vi "PI_Feedforward.vi"(5 "Motor Effort Axis":dbl[](array[numeric]) format="%_6g", 6 "dT":dbl, 7 "Position Axis":dbl[](array[numeric]) format="%_6g", 9 "Control Inputs":T2={"Kp"=0.01, "Ki"=0.0, "i upper"=0.0, "i lower"=0.0, "Output upper"=1.0, "Output lower"=-1.0}, 10 "Feed Back":dbl, 11 "Target":dbl) -> (1 "Term Indicators":T1, 2 "Output":dbl, 3 "Error":dbl)   [LabVIEW 2015]
uses:
  <vilib>/gmath/NI_Gmath.lvlib
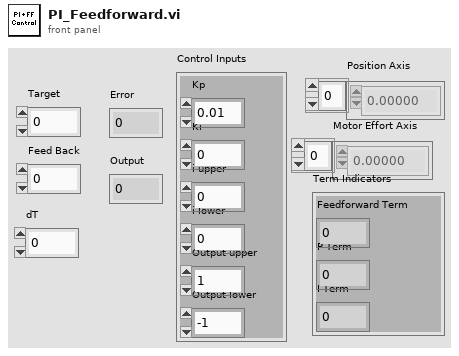
[diagram p1: front panel]
types:
  T1 = cluster{"Feedforward Term":dbl, "P Term ":dbl, "I Term":dbl}
  T2 = cluster{"Kp":dbl, "Ki":dbl, "i upper":dbl, "i lower":dbl, "Output upper":dbl, "Output lower":dbl}
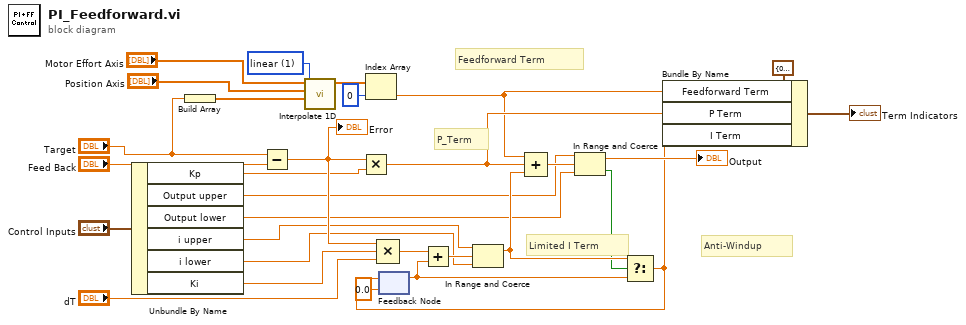
[diagram p0: block diagram]
diagram:
  w13 = 1 items=["nearest", "linear", "spline", "cubic Hermite", "Lagrange"] ("method")
  # "Feedforward Term"
  # "Anti-Windup"
  # "Limited I Term"
  # "P_Term"
  n1 = Unbundle By Name("Control Inputs") -> ("Kp"=w19:dbl, "Output upper"=w18:dbl, "Output lower"=w17:dbl, "i upper"=w16:dbl, "i lower"=w15:dbl, "Ki"=w14:dbl)
  n2 = Build Array("Target") -> (w11:dbl[])
  n3 = Subtract(x="Target", y="Feed Back") -> (x-y=w29:dbl)
  "Error" <- w29
  n4 = call <vilib>:"Interpolate 1D.vi"("method"=w13, "xi"=w11, "X"="Position Axis", "Y"="Motor Effort Axis") -> ("yi"=w8:dbl[])  [unwired: 5 in, 2 out]
  n5 = Multiply(x=w29, y=w19) -> (x*y=w4:dbl)
  n6 = Index Array(array=w8, index=0) -> (element=w2:dbl)
  n7 = Compound Arithmetic op=MULTIPLY(w29, w14, "dT") -> (w27:dbl)
  n8 = feedback #1(0.0 ("i upper")) -> (w22:dbl)
  n9 = Add(x=w27, y=w22) -> (x+y=w26:dbl)
  n10 = In Range and Coerce(upper limit=w16, x=w26, lower limit=w15) -> (coerced(x)=w23:dbl)  [unwired: 1 out]
  n11 = Compound Arithmetic op=ADD(w2, w4, w23) -> (w25:dbl)
  n12 = In Range and Coerce(upper limit=w18, x=w25, lower limit=w17) -> (coerced(x)=→"Output":dbl, In Range?=w21:bool)
  n13 = Select(t=w23, s=w21, f=w22) -> (s? t:f=w3:dbl)
  n14 = feedback-in #1(w3) -> ()
  n15 = Bundle By Name(cluster=T1 {"Feedforward Term"=0.0, "P Term "=0.0, "I Term"=0.0} ("Term Indicators"), "Feedforward Term"=w2, "P Term"=w4, "I Term"=w3) -> (→"Term Indicators":T1)
